vi "test7.vi"   [LabVIEW 2012, in "joystick.lvrbt"]
uses:
  joystick.lvrbt
  <vilib>/NXT/Hardware/Plugins/Tetrix DC Motor/TetrixDCMotorAddress.ctl
  <vilib>/NXT/Hardware/Plugins/Tetrix 180 deg Servo/Tetrix180ServoAddress.ctl
  <vilib>/FTC/FTC Read Controller Packet.vi
  <vilib>/FTC/FTC Interpret Motor Power From Right Y Axis.vi
  <vilib>/FTC/FTC Interpret Motor Power From Left Y Axis.vi
  <vilib>/NXT/NXTIO Xnodes/NXTIONodeSubVIs/TETRIX IO Move DC Motors.vi
  <vilib>/FTC/FTC Interpret Servo Position From Right Y Axis.vi
  <vilib>/NXT/NXTIO Xnodes/NXTIONodeSubVIs/TETRIX IO Move Servos.vi
  <vilib>/NXT/NXTIO Xnodes/NXTIONodeSubVIs/TETRIX IO Check Battery.vi
  <vilib>/NXT/NXTIO Xnodes/NXTIONodeSubVIs/TETRIX IO Stop DC Motors.vi
  <vilib>/NXT/Subs/LVHSConnector.ctl
  <vilib>/NXT/NXTIO Xnodes/AddressXNode/NXTIOAddress.xnode
  <vilib>/NXT/NXTIO Xnodes/NXTIOXNode/NXTIO.xnode
  <vilib>/NXT/LegoClasses/BrickReference/BrickReference.lvclass
panel:
  # "This VI was generated based on your configuration in the Remote Control Editor. You may modify the code as needed for your robot. To test this program for an FTC match, return to the Remote Control Editor, select the \"Run Program\" tab, and choose \"FTC Game\"."
types:
  T1 = typedef "TetrixDCMotorAddress.ctl" = i16
  T2 = cluster{"TetrixDCMotor":T1, "TetrixDCMotor 2":T1}
  T3 = typedef "LVHSConnector.ctl" = refnum<class "BrickReference.lvclass">
  T4 = typedef "FTC ControllerState.ctl" = cluster{"Left X":i8, "Left Y":i8, "Right X":i8, "Right Y":i8, "Button Encoding 9-12":u8, "Button Encoding 1-8":u8, "POV":T5}
  T5 = typedef "FTC POVState.ctl" = i8
  T6 = typedef "Tetrix180ServoAddress.ctl" = i16
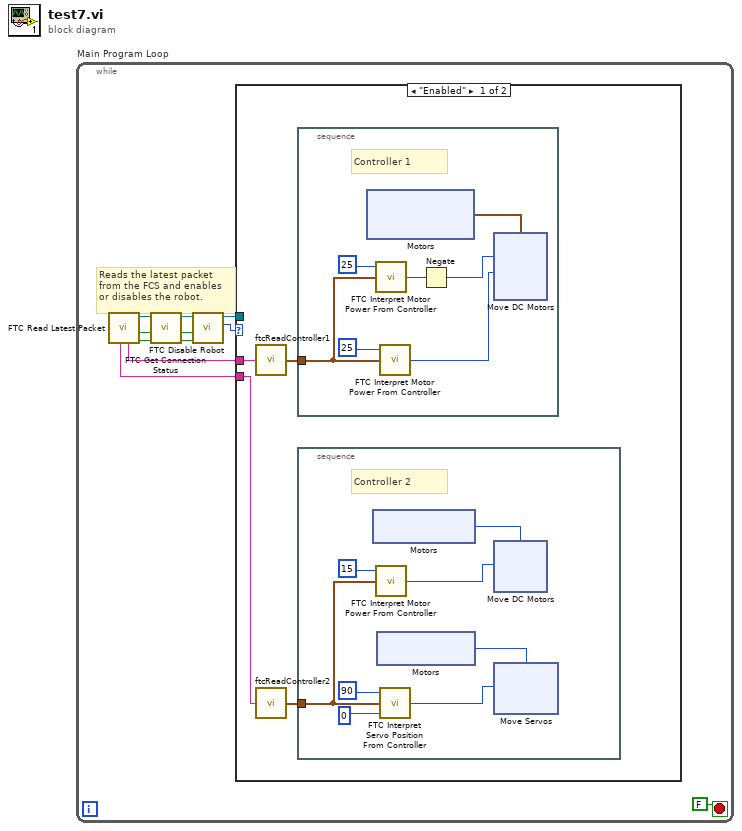
[diagram p0: block diagram]
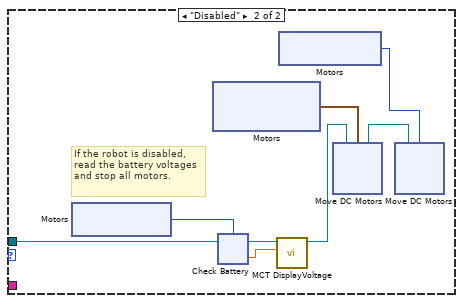
[diagram p2: hidden frame]
diagram:
  n1 = while "Main Program Loop" {
    stop <- FALSE stop-if-true
    # "Reads the latest packet\nfrom the FCS and enables\nor disables the robot."
    n2 = call <vilib>:"FTC Read Latest Packet.vi"() -> ("Packet Received?"=w8:bool, "Stopped?"=w5:bool, "NXT"=w7:T3, "Controller 1"=w10:string, "Controller 2"=w9:string)  [unwired: 6 in, 1 out]
    n3 = call <vilib>:"FTC Get Connection Status.vi"("Packet Received?"=w8, "Stopped?"=w5, "NXT"=w7) -> ("Online?"=w2:bool, "Stopped?"=w3:bool, "NXT"=w4:T3)  [unwired: 5 in]
    n4 = call <vilib>:"FTC Disable Robot.vi"("Online?"=w2, "Stopped?"=w3, "NXT"=w4) -> ("Enabled?"=w6:enum16{"Disabled", "Enabled"}, "NXT"=w1:T3)  [unwired: 3 in]
    n5 = case "disableCase" shown="\"Enabled\"" w6 {
      tunnel: w10 -> [w15 _]
      tunnel: w9 -> [w14 _]
      tunnel: w1 -> [_ w65]
      frame "Enabled" {
        n6 = call "ftcReadController1"("Packet"=w15) -> ("Controller State"=w13:T4)  [unwired: 4 in]
        n7 = call "ftcReadController2"("Packet"=w14) -> ("Controller State"=w12:T4)  [unwired: 4 in]
        n8 = stacked-sequence "controller1Actions" {
          tunnel: w13 -> [w46]
          frame #0 {
            # "Controller 1"
            n9 = xnode ("Motors")() -> ("Motor"=w44:cluster{"TetrixDCMotor":T1, "TetrixDCMotor":T1})
            n10 = call-poly <vilib>:"FTC Interpret Motor Power From Controller.vi"("Controller State"=w46, "Power Level (50)"=i8 25) -> ("Power"=w43:i8)  [unwired: 1 in]
            n11 = call-poly <vilib>:"FTC Interpret Motor Power From Controller.vi"("Controller State"=w46, "Power Level (50)"=i8 25) -> ("Power"=w41:i8)  [unwired: 1 in]
            n12 = Negate(x=w43) -> (-x=w40:i8)
            n13 = xnode ("Move DC Motors")("Power/Speed 2"=w41, "Power/Speed 1"=w40, "Motors"=w44) -> ()  [unwired: 1 in, 1 out]
          }
        }
        n14 = stacked-sequence "controller2Actions" {
          tunnel: w12 -> [w23]
          frame #0 {
            # "Controller 2"
            n15 = xnode ("Motors")() -> ("Motor"=w21:T1)
            n16 = call-poly <vilib>:"FTC Interpret Motor Power From Controller.vi"("Controller State"=w23, "Power Level (50)"=i8 15) -> ("Power"=w20:i8)  [unwired: 1 in]
            n17 = xnode ("Motors")() -> ("Motor"=w17:T6)
            n18 = call-poly <vilib>:"FTC Interpret Servo Position From Controller.vi"("Lower Limit (0)"=i16 0, "Controller State"=w23, "Upper Limit (255)"=i16 90) -> ("Position"=w16:u8)
            n19 = xnode ("Move DC Motors")("Power/Speed 1"=w20, "Motors"=w21) -> ()  [unwired: 1 in, 1 out]
            n20 = xnode ("Move Servos")("Position 1"=w16, "Servos"=w17) -> ()  [unwired: 1 in, 1 out]
          }
        }
      }
      frame "Disabled" {
        # "If the robot is disabled, read the battery voltages and stop all motors."
        n21 = xnode ("Motors")() -> ("Motor"=w64:T1)
        n22 = xnode "Motors"() -> ("Motor"=w61:cluster{"TetrixDCMotor":T1, "TetrixDCMotor":T1})
        n23 = xnode ("Check Battery")("Motors"=w64, "NXT"=w65) -> ("Voltage 1"=w63:sgl, "NXT"=w62:T3)
        n24 = call <vilib>:"MCT DisplayVoltage.vi"("Motor Voltage"=w63, "NXT"=w62) -> ("NXT"=w60:T3)  [unwired: 9 in]
        n25 = xnode "Motors"() -> ("Motor"=w59:T1)
        n26 = xnode "Move DC Motors"("Motors"=w61, "NXT"=w60) -> ("NXT"=w58:T3)
        n27 = xnode "Move DC Motors"("Motors"=w59, "NXT"=w58) -> ()  [unwired: 1 out]
      }
    }
  }
